vi "Sending and Receive U32 CMD and Data.vi"(0 "TCP Ref In":refnum<k5>, 1 "Time Out(ms)":i32=100, 5 "CMD In":u32 format="%.0x", 7 "Data In":string, 11 "error in (no error)":errorcluster) -> (4 "TCP Ref Out":refnum<k5>, 6 "CMD Out":u32 format="%.0x", 8 "Data Out":string, 15 "error out":errorcluster)   [LabVIEW 2024]
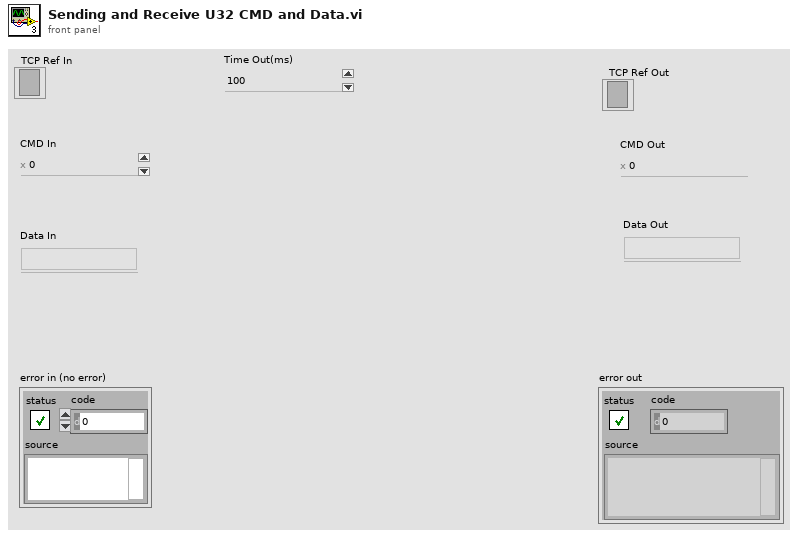
[diagram p1: front panel]
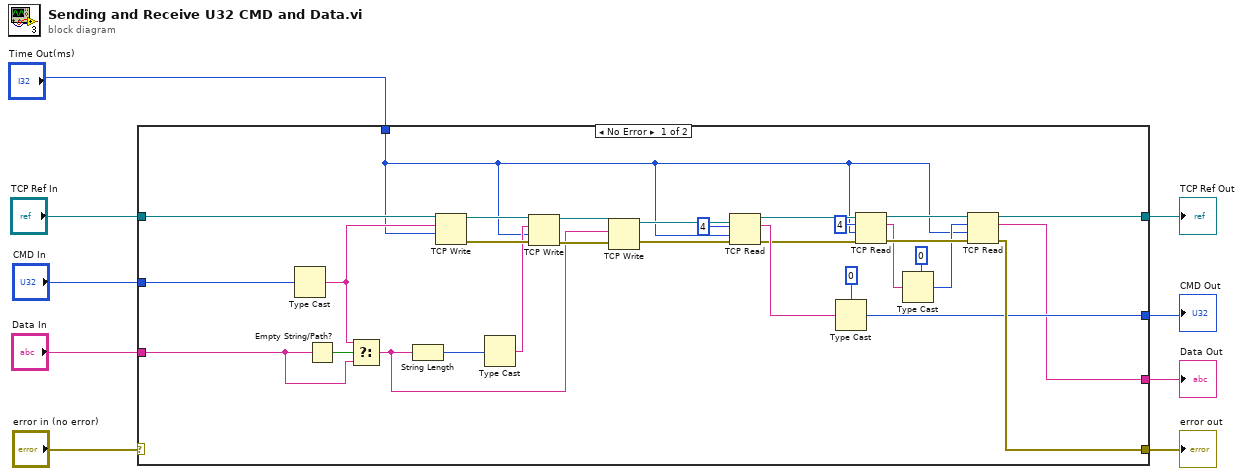
[diagram p0: block diagram]
diagram:
  n1 = case shown="No Error" "error in (no error)" {
    selector: "error in (no error)" -> [_ w41]
    tunnel: [w12 w41] -> w8
    tunnel: "Data In" -> [w32 _]
    tunnel: "CMD In" -> [w30 _]
    tunnel: "TCP Ref In" -> [w31 w40]
    tunnel: [w17 w40] -> w4
    tunnel: "Time Out(ms)" -> [w13 _]
    tunnel: [w11 _] -> w2
    tunnel: [w10 _] -> w1
    frame No Error {
      n2 = Type Cast(x=w30) -> (*(type *) &x=w34:string)  [unwired: 1 in]
      n3 = Empty String/Path?(string/path=w32) -> (empty?=w35:bool)
      n4 = Select(t=w34, s=w35, f=w32) -> (s? t:f=w33:string)
      n5 = String Length(string=w33) -> (length=w29:i32)
      n6 = TCP Write(connection ID=w31, data in=w34, 9:w13) -> (connection ID out=w39:refnum<k5>, error out=w38:errorcluster)  [unwired: 1 in, 1 out]
      n7 = Type Cast(x=w29) -> (*(type *) &x=w36:string)  [unwired: 1 in]
      n8 = TCP Write(connection ID=w39, data in=w36, error in (no error)=w38, 9:w13) -> (connection ID out=w16:refnum<k5>, error out=w37:errorcluster)  [unwired: 1 out]
      n9 = TCP Write(connection ID=w16, data in=w33, error in (no error)=w37) -> (connection ID out=w15:refnum<k5>, error out=w14:errorcluster)  [unwired: 1 in, 1 out]
      n10 = TCP Read(connection ID=w15, bytes to read=4, error in (no error)=w14, 9:w13) -> (connection ID out=w27:refnum<k5>, data out=w26:string, error out=w24:errorcluster)  [unwired: 1 in]
      n11 = Type Cast(type=u32 0 ("bytes to read"), x=w26) -> (*(type *) &x=w11:u32)
      n12 = TCP Read(connection ID=w27, bytes to read=4, error in (no error)=w24, 9:w13) -> (connection ID out=w21:refnum<k5>, data out=w19:string, error out=w22:errorcluster)  [unwired: 1 in]
      n13 = Type Cast(type=0 ("bytes to read"), x=w19) -> (*(type *) &x=w18:i32)
      n14 = TCP Read(connection ID=w21, bytes to read=w18, error in (no error)=w22, 9:w13) -> (connection ID out=w17:refnum<k5>, data out=w10:string, error out=w12:errorcluster)  [unwired: 1 in]
    }
    frame Error {
    }
  }
  "error out" <- w8
  "TCP Ref Out" <- w4
  "CMD Out" <- w2
  "Data Out" <- w1
